vi "Read Name Dependecy.vi"(8 "error in (no error)":errorcluster, 11 "Listbox TBDT in":refnum<class "Listbox TBDT.lvclass">) -> (0 "error out":errorcluster, 2 "Name Dependecy":i32, 3 "Listbox TBDT out":refnum<class "Listbox TBDT.lvclass">)   [LabVIEW 2013, in "Table Manager.lvlib" / "Listbox TBDT.lvclass"]
uses:
  Listbox TBDT.lvclass
  Listbox TBDT.lvclass/Listbox TBDT.ctl
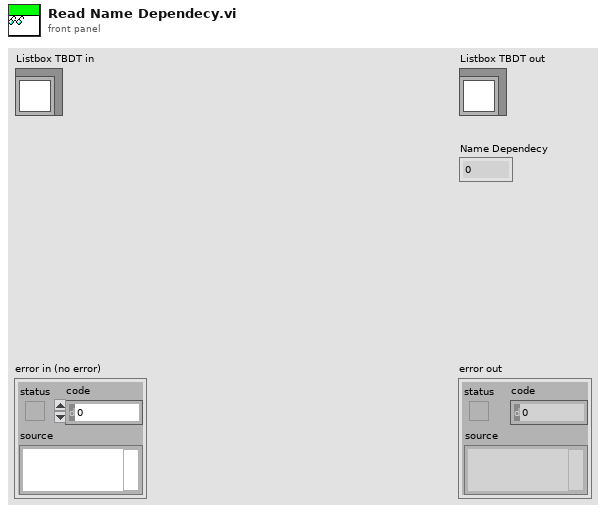
[diagram p1: front panel]
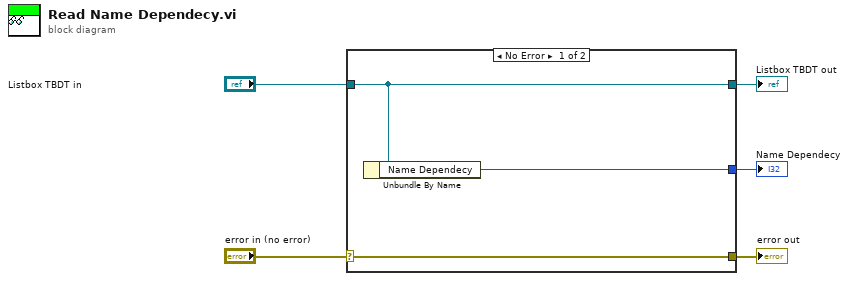
[diagram p0: block diagram]
diagram:
  n1 = case shown="No Error" "error in (no error)" {
    selector: "error in (no error)" -> [w8 w9]
    tunnel: [w8 w9] -> w4
    tunnel: [w7 w10] -> w2
    tunnel: "Listbox TBDT in" -> [w7 w10]
    tunnel: [w6 _] -> w1
    frame No Error {
      n2 = Unbundle By Name(w7) -> ("Name Dependecy"=w6:i32)
    }
    frame Error {
    }
  }
  "error out" <- w4
  "Listbox TBDT out" <- w2
  "Name Dependecy" <- w1
